vi "Steps Handler.vi"(7 "Operation":enum16{"Setup", "Next State"}(ring), 10 "Wash Options":T2) -> (2 "Next State":T1)   [LabVIEW 2025]
uses:
  Controls/Controls.ctl
  Controls/Wash Options.ctl
panel:
  in  "States":T1
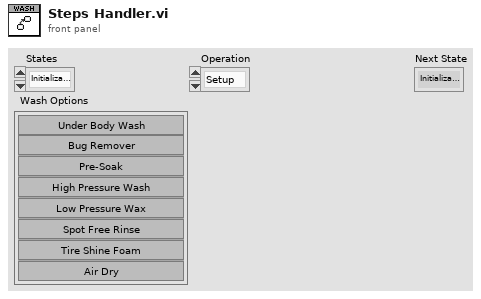
[diagram p1: front panel]
types:
  T1 = typedef "Controls.ctl" = enum16{"Initialization", "Wait For Start", "Car Wash Setup", "Under Body Wash", "Bug Remover", "Pre-Soak", "High Pressure Wash", "Low Pressure Wash", "Spot Free Rinse", "Tire Shine Foam", "Air Dry", "Exit"}
  T2 = typedef "Wash Options.ctl" = cluster{"Underbody Wash":bool, "Bug Remover":bool, "Pre-Soak":bool, "High Pressure Wash":bool, "Low Pressure Wax":bool, "Spot Free Rinse":bool, "Tire Shine Foam":bool, "Air Dry":bool}
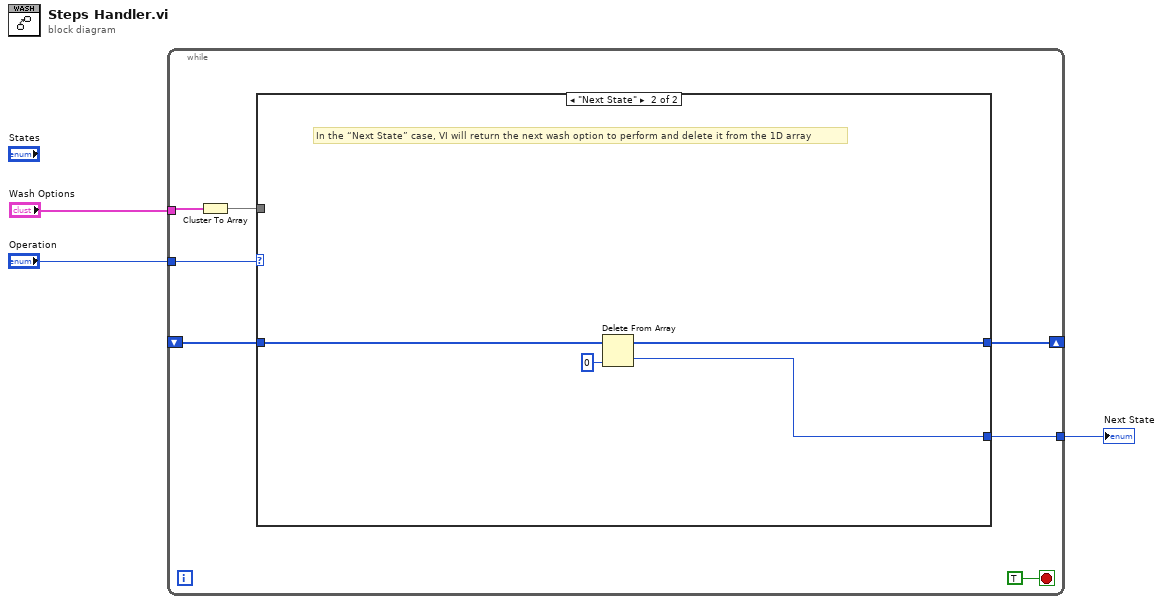
[diagram p0: block diagram]
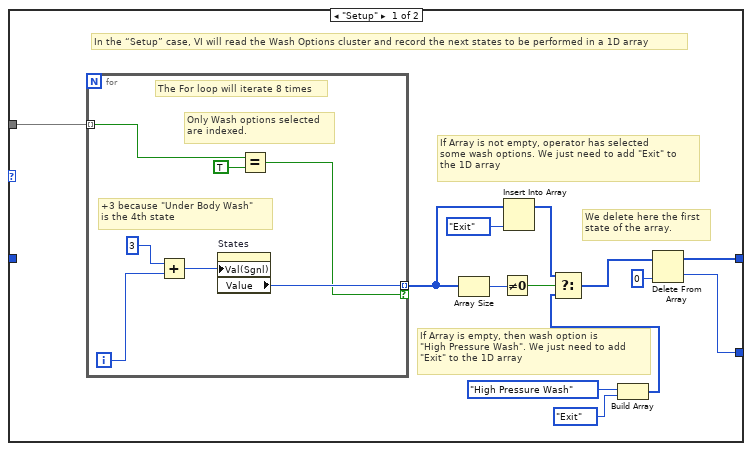
[diagram p2: hidden frame]
diagram:
  n1 = while {
    tunnel: "Operation" -> [w10]
    tunnel: "Wash Options" -> [w9]
    tunnel: [w6] -> w1
    shift-right: [w7] -> _
    shift-left: _ -> [w5]
    stop <- TRUE stop-if-true
    n2 = Cluster To Array(cluster=w9) -> (array=w8:bool[])
    n3 = case shown="\"Next State\"" w10 {
      tunnel: w8 -> [w23 _]
      tunnel: [w13 w33] -> w7
      tunnel: [w12 w31] -> w6
      tunnel: w5 -> [_ w34]
      frame "Setup" {
        # "We delete here the first \nstate of the array."
        # "If Array is empty, then wash option is \n\"High Pressure Wash\". We just need to add \n\"Exit\" to the 1D array"
        # "If Array is not empty, operator has selected\nsome wash options. We just need to add \"Exit\" to\nthe 1D array"
        # "In the “Setup” case, VI will read the Wash Options cluster and record the next states to be performed in a 1D array"
        n4 = for {
          tunnel: w23 -> [w26] mode=indexing
          tunnel: [w27] -> w20 mode=indexing if=w24
          i -> [w30]
          # "Only Wash options selected\nare indexed."
          # "+3 because \"Under Body Wash\" \nis the 4th state"
          # "The For loop will iterate 8 times"
          n5 = Add(x=3, y=w30) -> (x+y=w28:i32)
          n6 = property on="States" class="Enum (strict)"("Val(Sgnl)"=w28) -> ("Value"=w27:T1)  [unwired: 2 in, 2 out]
          n7 = Equal?(x=w26, y=TRUE) -> (x = y?=w24:bool)
        }
        n8 = Array Size(array=w20) -> (size(s)=w22:i32)
        n9 = Not Equal To 0?(x=w22) -> (x != 0?=w21:bool)
        n10 = Insert Into Array(array=w20, new element=Controls."Exit" ("new element/subarray")) -> (w19:T1[])  [unwired: 1 in]
        n11 = Build Array(Controls."High Pressure Wash" ("new element/subarray"), Controls."Exit" ("new element/subarray")) -> (w15:T1[])
        n12 = Select(t=w19, s=w21, f=w15) -> (s? t:f=w14:T1[])
        n13 = Delete From Array(array=w14, index=0) -> (deleted portion=w12:T1, array with subset deleted=w13:T1[])  [unwired: 1 in]
      }
      frame "Next State" {
        # "In the “Next State” case, VI will return the next wash option to perform and delete it from the 1D array"
        n14 = Delete From Array(array=w34, index=0) -> (deleted portion=w31:T1, array with subset deleted=w33:T1[])  [unwired: 1 in]
      }
    }
  }
  "Next State" <- w1
